vi "getFactory.vi"(8 "error in (no error)":errorcluster, 10 "choice":string, 11 "FactoryProducer in":refnum<class "FactoryProducer.lvclass">) -> (0 "error out":errorcluster, 2 "AbstractFactory":refnum<class "AbstractFactory.lvclass">, 3 "FactoryProducer out":refnum<class "FactoryProducer.lvclass">)   [LabVIEW 2018, in "FactoryProducer.lvclass"]
uses:
  FactoryProducer.lvclass
  AbstractFactory Class/AbstractFactory.lvclass
  ShapeFactory Class/ShapeFactory.lvclass
  C:/Users/fflores/Documents/LabVIEW-Open-Projects/LabIVEW OOP Design Patterns/Abstract Factory Pattern/AbstractFactory Class/AbstractFactory.lvclass
  ColorFactory Class/ColorFactory.lvclass
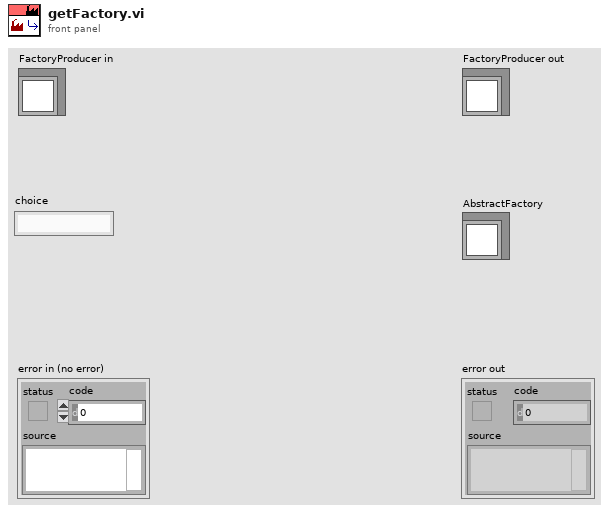
[diagram p1: front panel]
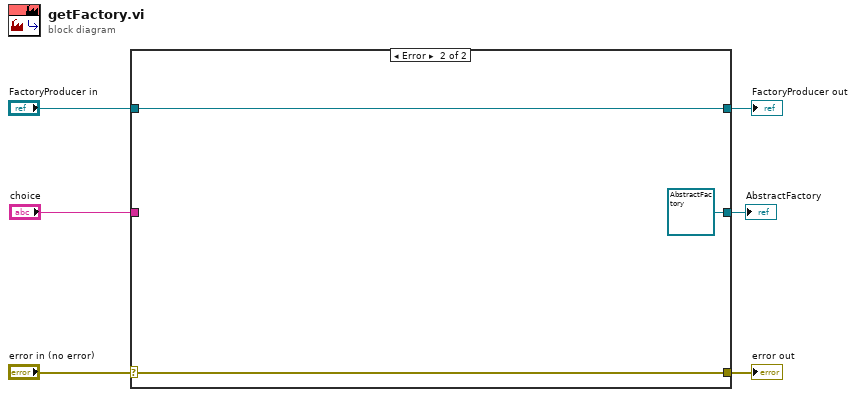
[diagram p0: block diagram]
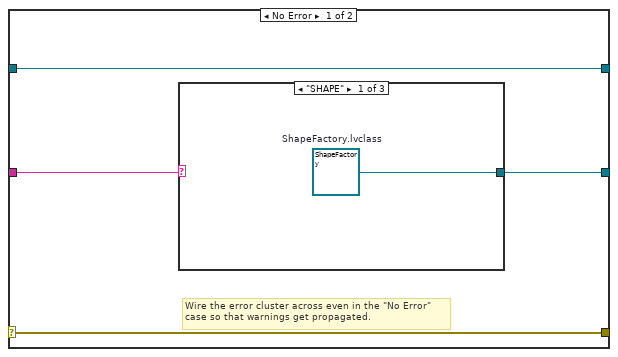
[diagram p2: hidden frame]
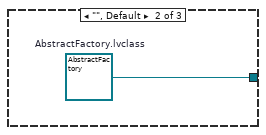
[diagram p3: hidden frame]
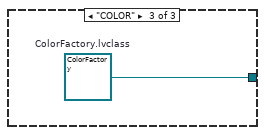
[diagram p4: hidden frame]
diagram:
  n1 = case shown="Error" "error in (no error)" {
    selector: "error in (no error)" -> [w9 w16]
    tunnel: [w9 w16] -> w5
    tunnel: [w10 w15] -> w3
    tunnel: "FactoryProducer in" -> [w10 w15]
    tunnel: "choice" -> [w8 _]
    tunnel: [w7 refnum<class "AbstractFactory.lvclass"> refnum ("AbstractFactory.lvclass")] -> w1
    frame No Error {
      # "Wire the error cluster across even in the \"No Error\"\ncase so that warnings get propagated."
      n2 = case shown="\"SHAPE\"" w8 {
        tunnel: [w11 w12 w13] -> w7
        frame "SHAPE" {
          w11 = refnum<class "ShapeFactory.lvclass"> refnum  # ShapeFactory.lvclass
        }
        frame "", Default {
          w12 = refnum<class "AbstractFactory.lvclass"> refnum  # AbstractFactory.lvclass
        }
        frame "COLOR" {
          w13 = refnum<class "ColorFactory.lvclass"> refnum  # ColorFactory.lvclass
        }
      }
    }
    frame Error {
    }
  }
  "error out" <- w5
  "FactoryProducer out" <- w3
  "AbstractFactory" <- w1
